vi "mag-field_perm-mode_ramp.vi"(9 "actual field":dbl, 10 "goto field":dbl, 11 "GPIB adr in":string) -> ()   [LabVIEW 2010]
panel:
  in  "emergency stop":bool
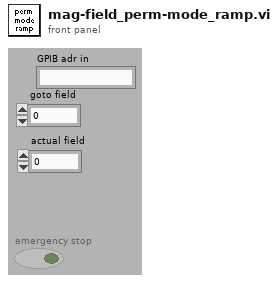
[diagram p1: front panel]
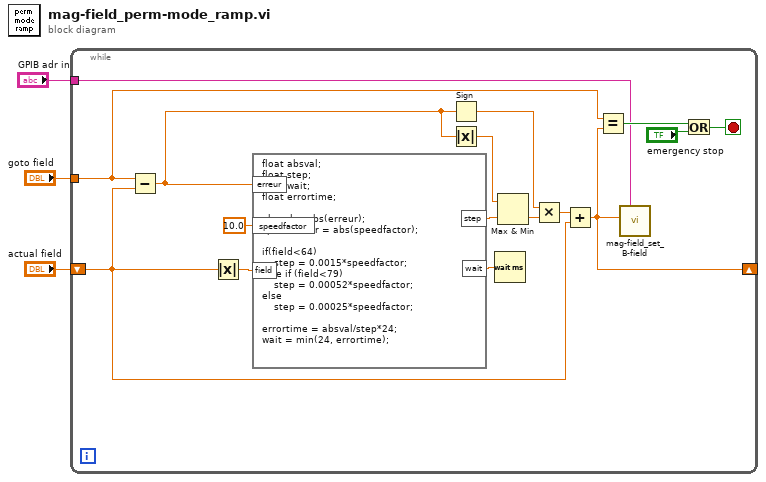
[diagram p0: block diagram]
diagram:
  n1 = while {
    shift-right: [w5] -> _
    shift-left: "actual field" -> [w12]
    tunnel: "goto field" -> [w4]
    tunnel: "GPIB adr in" -> [w10]
    stop <- w9 stop-if-true
    n2 = Subtract(x=w4, y=w12) -> (x-y=w6:dbl)
    n3 = Absolute Value(x=w12) -> (abs(x)=w15:dbl)
    n4 = formula code="float absval;\nfloat step;\nfloat wait;\nfloat errortime;\n\nabsval = abs(erreur);\nspeedfactor = abs(speedfactor);\n\nif(field<64)\n    step = 0.0015*speedfactor;\nelse if (field<79)\n    step = 0.00052*speedfactor;\nelse\n    step = 0.00025*speedfactor;\n\nerrortime = absval/step*24;\nwait = min(24, errortime);"("field"=w15, "erreur"=w6, "speedfactor"=10.0 ("input variable")) -> ("step"=w18:dbl, "wait"=w13:dbl)
    n5 = Sign(1:w6) -> (0:w14:dbl)
    n6 = Absolute Value(x=w6) -> (abs(x)=w19:dbl)
    n7 = Wait (ms)(milliseconds to wait=w13) -> ()  [unwired: 1 out]
    n8 = Max & Min(x=w19, y=w18) -> (min(x,y)=w17:dbl)  [unwired: 1 out]
    n9 = Multiply(x=w14, y=w17) -> (x*y=w16:dbl)
    n10 = Add(x=w16, y=w12) -> (x+y=w5:dbl)
    n11 = Equal?(x=w4, y=w5) -> (x = y?=w11:bool)
    n12 = call "mag-field_set_B-field.vi"("Field (T)"=w5, "GPIB adr in"=w10) -> ()  [unwired: 10 out]
    n13 = Or(x=w11, y="emergency stop") -> (x .or. y?=w9:bool)
  }
